vi "json字符串.vi"   [LabVIEW 2020]
uses:
  <vilib>/addons/_JKI.lib/Serialization/JSON/JKI JSON Serialization.lvlib
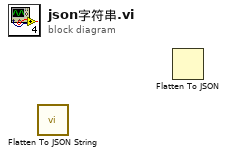
[diagram p0: block diagram]
diagram:
  n1 = call <vilib>:"Flatten To JSON String.vi"() -> ()  [unwired: 10 in, 2 out]
  n2 = Flatten To JSON() -> ()  [unwired: 3 in, 2 out]
